vi "Write Denuded.vi"(8 "error in (no error)":errorcluster, 10 "Denuded":bool, 11 "ePAS Data in":refnum<class "ePAS Data.lvclass">) -> (0 "error out":errorcluster, 3 "ePAS Data out":refnum<class "ePAS Data.lvclass">)   [LabVIEW 2014, in "ePAS Data.lvclass"]
uses:
  ePAS Data.lvclass
  ePAS Data.lvclass/ePAS Data.ctl
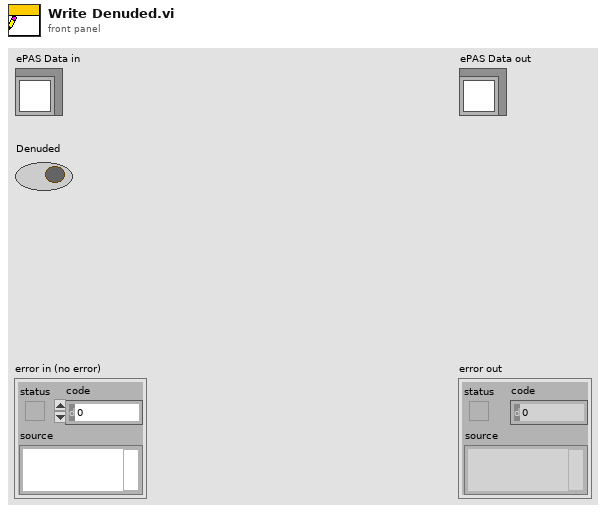
[diagram p1: front panel]
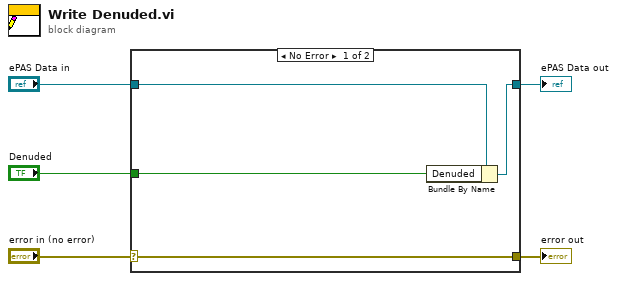
[diagram p0: block diagram]
diagram:
  n1 = case shown="No Error" "error in (no error)" {
    selector: "error in (no error)" -> [w9 w10]
    tunnel: [w9 w10] -> w4
    tunnel: [w7 w11] -> w2
    tunnel: "ePAS Data in" -> [w8 w11]
    tunnel: "Denuded" -> [w6 _]
    frame No Error {
      n2 = Bundle By Name(cluster=w8, "Denuded"=w6) -> (w7:refnum<class "ePAS Data.lvclass">)
    }
    frame Error {
    }
  }
  "error out" <- w4
  "ePAS Data out" <- w2
